vi "Write Element of dI_dV.vi"(8 "error in (no error)":errorcluster, 9 "Numeric":dbl, 10 "index":i32, 11 "IV_data in":refnum<class "IV_data.lvclass">) -> (0 "error out":errorcluster, 3 "IV_data out":refnum<class "IV_data.lvclass">)   [LabVIEW 2014, in "IV_data.lvclass"]
uses:
  IV_data.lvclass
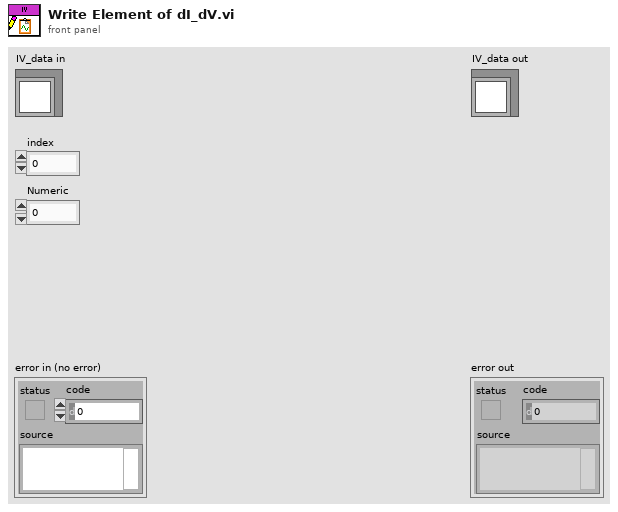
[diagram p1: front panel]
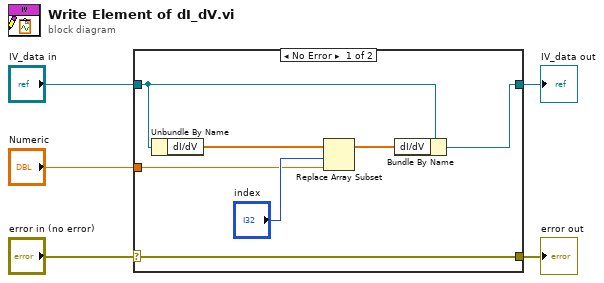
[diagram p0: block diagram]
diagram:
  n1 = case shown="No Error" "error in (no error)" {
    selector: "error in (no error)" -> [w12 w13]
    tunnel: [w12 w13] -> w4
    tunnel: [w11 w14] -> w2
    tunnel: "IV_data in" -> [w10 w14]
    tunnel: "Numeric" -> [w6 _]
    frame No Error {
      n2 = Unbundle By Name(w10) -> ("dI/dV"=w9:dbl[])
      n3 = Replace Array Subset(array=w9, new element=w6, index="index") -> (w8:dbl[])
      n4 = Bundle By Name(cluster=w10, "dI/dV"=w8) -> (w11:refnum<class "IV_data.lvclass">)
    }
    frame Error {
    }
  }
  "error out" <- w4
  "IV_data out" <- w2
